vi "Change Count.vi"(0 "connection ID in":refnum<k5>, 2 "Timeout (ms)":i32=40000000, 3 "TxFreqIndex":i32, 4 "TxWaveformStyle":i32, 5 "TxFreqIndex":dbl[](array[numeric])) -> (7 "connection ID out":refnum<k5>)   [LabVIEW 2016]
uses:
  TemperatureMeasure/Thermal_type.vi
panel:
  out "Matched Txfreq":i32[](array[numeric])
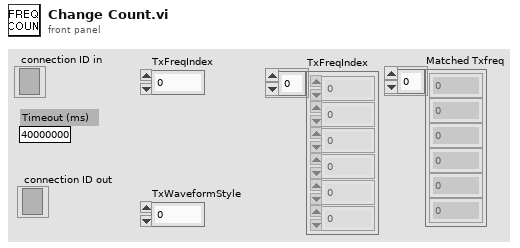
[diagram p1: front panel]
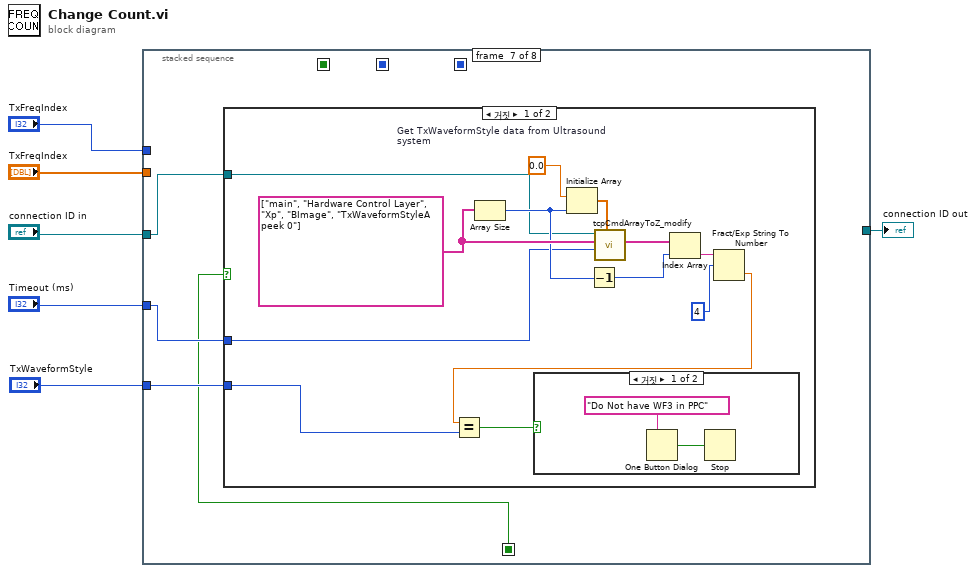
[diagram p0: block diagram]
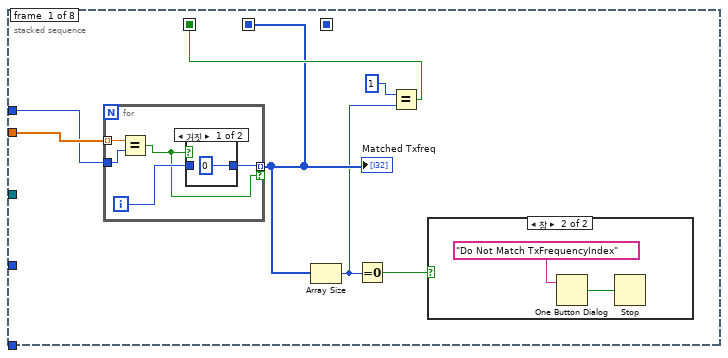
[diagram p2: hidden frame]
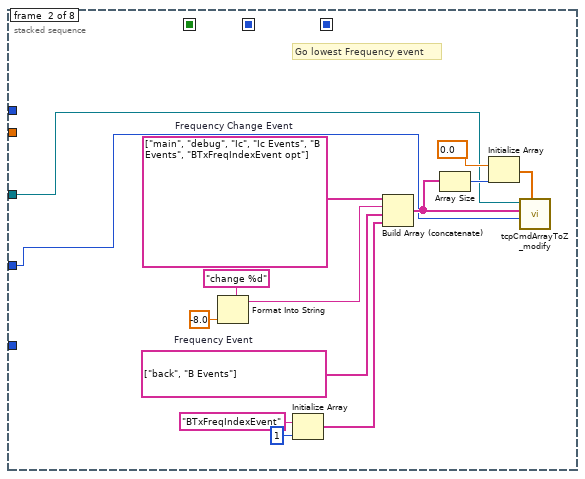
[diagram p5: hidden frame]
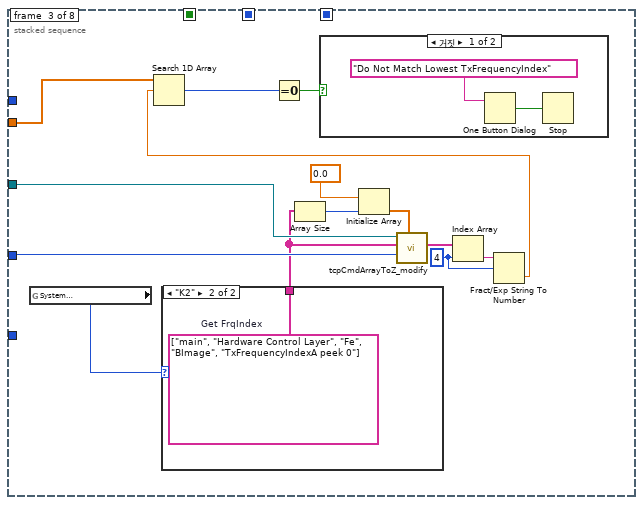
[diagram p6: hidden frame]
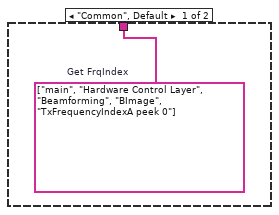
[diagram p7: hidden frame]
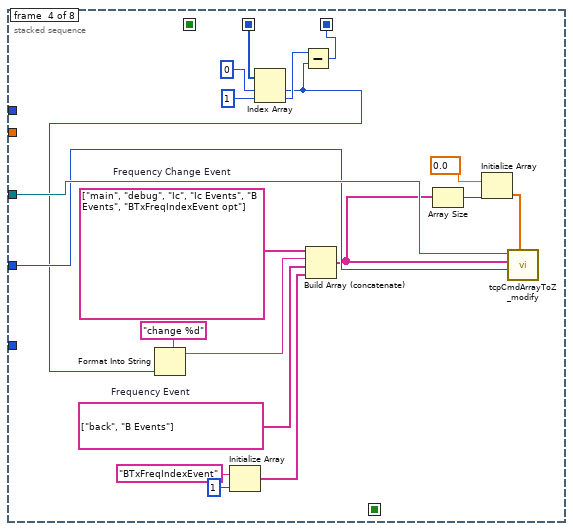
[diagram p9: hidden frame]
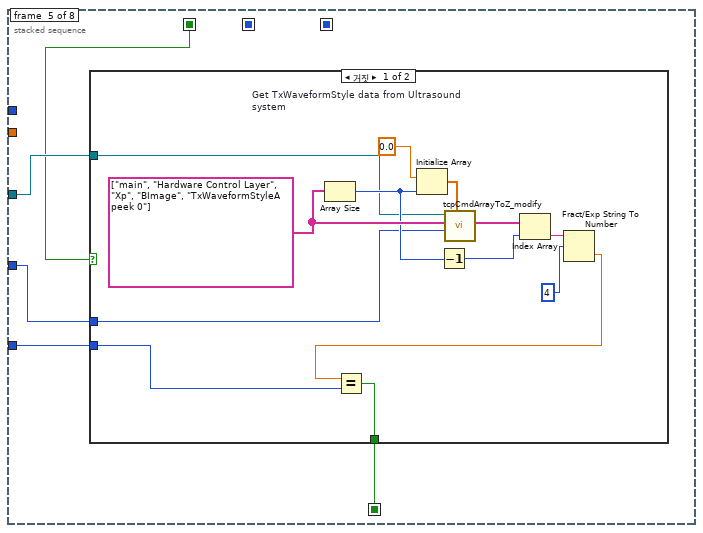
[diagram p10: hidden frame]
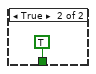
[diagram p11: hidden frame]
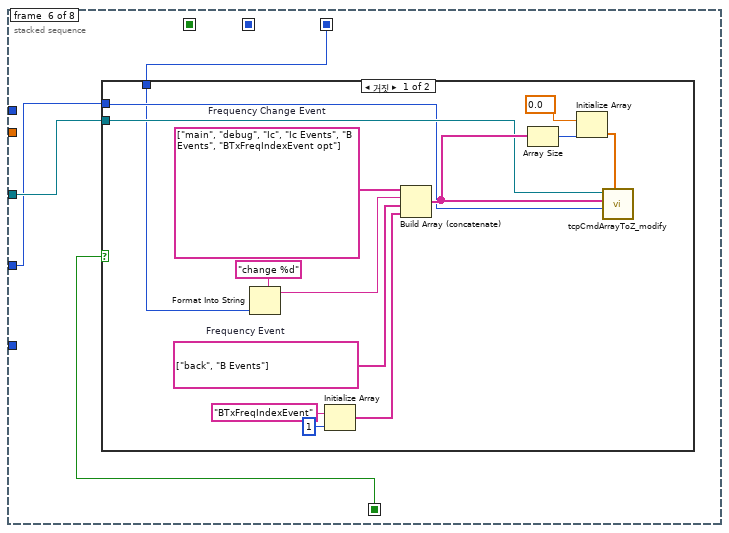
[diagram p12: hidden frame]
diagram:
  n1 = stacked-sequence {
    seq-local: [w10 _ _ _ _ _ _ _] -> [_ _ _ _ w76 _ _ _]
    seq-local: [w8 _ _ _ _ _ _ _] -> [_ _ _ w71 _ _ _ _]
    seq-local: [_ _ _ w56 _ _ _ _] -> [_ _ _ _ _ w94 _ _]
    seq-local: [_ _ _ _ w74 _ _ _] -> [_ _ _ _ _ w93 w112 _]
    tunnel: "TxFreqIndex" -> [w13 _ w42 _ _ _ _ _]
    tunnel: "TxFreqIndex" -> [w12 _ _ _ _ _ _ _]
    tunnel: "Timeout (ms)" -> [_ w24 w43 w72 w77 w95 w113 _]
    tunnel: "connection ID in" -> [_ w25 w44 w73 w78 w96 w111 w130]
    tunnel: [_ _ _ _ _ _ _ w130] -> w2
    tunnel: "TxWaveformStyle" -> [_ _ _ _ w75 _ w114 _]
    frame #0 {
      n2 = for {
        tunnel: w13 -> [w18] mode=indexing
        tunnel: w12 -> [w17]
        tunnel: [w16] -> w8 mode=indexing if=w14
        i -> [w15]
        n3 = Equal?(x=w18, y=w17) -> (x = y?=w14:bool)
        n4 = case shown="거짓" w14 {
          tunnel: [0 w20] -> w16
          tunnel: w15 -> [_ w20]
          frame False {
          }
          frame True {
          }
        }
      }
      "Matched Txfreq" <- w8
      n5 = Array Size(array=w8) -> (size(s)=w7:i32)
      n6 = Equal To 0?(x=w7) -> (x = 0?=w9:bool)
      n7 = Equal?(x=1, y=w7) -> (x = y?=w10:bool)
      n8 = case shown="참" w9 {
        frame False {
        }
        frame True {
          n9 = One Button Dialog(message="Do Not Match TxFrequencyIndex" ("메시지")) -> (true=w21:bool)  [unwired: 1 in]
          n10 = Stop(stop? (T)=w21) -> ()
        }
      }
    }
    frame #1 {
      w27 = string[] ["back", "B Events"]  # Frequency Event
      w31 = string[] ["main", "debug", "Ic", "Ic Events", "B Events", "BTxFreqIndexEvent opt"]  # Frequency Change Event
      # "Go lowest Frequency event"
      n11 = Format Into String(format string="change %d" ("Format String"), -8.0 ("입력 1")) -> (resulting string=w30:string)  [unwired: 2 in, 1 out]
      n12 = Initialize Array("BTxFreqIndexEvent", 1 ("dimension size")) -> (w26:string[])
      n13 = Build Array (concatenate)(w31, w30, w27, w26) -> (w34:string[])
      n14 = Array Size(array=w34) -> (size(s)=w36:i32)
      n15 = Initialize Array(sgl 0.0 ("element"), w36) -> (w33:sgl[])
      n16 = call "tcpCmdArrayToZ_modify.vi"("Delay (sec)"=w33, "Timeout (ms)"=w24, "Command array"=w34, "connection ID in"=w25) -> ()  [unwired: 3 in, 5 out]
    }
    frame #2 {
      w50 = 4 ("index")
      n17 = global read "Thermal_type.vi" "System \nSelection"() -> (w38:enum32{"Common", "Frosk", "Griffin", "K2"})
      n18 = case shown="\"K2\"" w38 {
        tunnel: [w51 w52] -> w37
        frame "Common", Default {
          w51 = string[] ["main", "Hardware Control Layer", "Beamforming", "BImage", "TxFrequencyIndexA peek 0"]  # Get FrqIndex
        }
        frame "K2" {
          w52 = string[] ["main", "Hardware Control Layer", "Fe", "BImage", "TxFrequencyIndexA peek 0"]  # Get FrqIndex
        }
      }
      n19 = Array Size(array=w37) -> (size(s)=w45:i32)
      n20 = Initialize Array(sgl 0.0 ("element"), w45) -> (w47:sgl[])
      n21 = call "tcpCmdArrayToZ_modify.vi"("Delay (sec)"=w47, "Timeout (ms)"=w43, "Command array"=w37, "connection ID in"=w44) -> ("Receive array"=w48:string[])  [unwired: 3 in, 4 out]
      n22 = Index Array(array=w48, index=w50) -> (element=w49:string)
      n23 = Fract/Exp String To Number(string=w49, offset=w50) -> (number=w41:dbl)  [unwired: 2 in, 1 out]
      n24 = Search 1D Array(1D array=w42, element=w41) -> (index of element=w39:i32)  [unwired: 1 in]
      n25 = Equal To 0?(x=w39) -> (x = 0?=w40:bool)
      n26 = case shown="거짓" w40 {
        frame False {
          n27 = One Button Dialog(message="Do Not Match Lowest TxFrequencyIndex" ("메시지")) -> (true=w53:bool)  [unwired: 1 in]
          n28 = Stop(stop? (T)=w53) -> ()
        }
        frame True {
        }
      }
    }
    frame #3 {
      w60 = string[] ["back", "B Events"]  # Frequency Event
      w64 = string[] ["main", "debug", "Ic", "Ic Events", "B Events", "BTxFreqIndexEvent opt"]  # Frequency Change Event
      n29 = Initialize Array("BTxFreqIndexEvent", 1 ("dimension size")) -> (w59:string[])
      n30 = Index Array(array=w71, index #1=0 ("인덱스"), index #2=1 ("인덱스")) -> (element #1=w55:i32, element #2=w57:i32)
      n31 = Format Into String(format string="change %d" ("Format String"), w55) -> (resulting string=w63:string)  [unwired: 2 in, 1 out]
      n32 = Subtract(x=w57, y=w55) -> (x-y=w56:i32)
      n33 = Build Array (concatenate)(w64, w63, w60, w59) -> (w67:string[])
      n34 = Array Size(array=w67) -> (size(s)=w69:i32)
      n35 = Initialize Array(sgl 0.0 ("element"), w69) -> (w66:sgl[])
      n36 = call "tcpCmdArrayToZ_modify.vi"("Delay (sec)"=w66, "Timeout (ms)"=w72, "Command array"=w67, "connection ID in"=w73) -> ()  [unwired: 3 in, 5 out]
    }
    frame #4 {
      n37 = case shown="거짓" w76 {
        tunnel: w78 -> [w83 _]
        tunnel: w77 -> [w82 _]
        tunnel: w75 -> [w81 _]
        tunnel: [w79 TRUE] -> w74
        frame False {
          w91 = string[] ["main", "Hardware Control Layer", "Xp", "BImage", "TxWaveformStyleA peek 0"]  # Get TxWaveformStyle data from Ultrasound system
          n38 = Array Size(array=w91) -> (size(s)=w87:i32)
          n39 = Initialize Array(0.0 ("원소"), w87) -> (w89:dbl[])
          n40 = Decrement(x=w87) -> (x-1=w85:i32)
          n41 = call "tcpCmdArrayToZ_modify.vi"("Delay (sec)"=w89, "Timeout (ms)"=w82, "Command array"=w91, "connection ID in"=w83) -> ("Receive array"=w88:string[])  [unwired: 3 in, 4 out]
          n42 = Index Array(array=w88, index=w85) -> (element=w86:string)
          n43 = Fract/Exp String To Number(string=w86, offset=4 ("오프셋")) -> (number=w80:dbl)  [unwired: 2 in, 1 out]
          n44 = Equal?(x=w80, y=w81) -> (x = y?=w79:bool)
        }
        frame True {
        }
      }
    }
    frame #5 {
      n45 = case shown="거짓" w93 {
        tunnel: w96 -> [w99 _]
        tunnel: w95 -> [w98 _]
        tunnel: w94 -> [w97 _]
        frame False {
          w101 = string[] ["back", "B Events"]  # Frequency Event
          w105 = string[] ["main", "debug", "Ic", "Ic Events", "B Events", "BTxFreqIndexEvent opt"]  # Frequency Change Event
          n46 = Format Into String(format string="change %d" ("Format String"), w97) -> (resulting string=w104:string)  [unwired: 2 in, 1 out]
          n47 = Initialize Array("BTxFreqIndexEvent", 1 ("dimension size")) -> (w100:string[])
          n48 = Build Array (concatenate)(w105, w104, w101, w100) -> (w108:string[])
          n49 = Array Size(array=w108) -> (size(s)=w110:i32)
          n50 = Initialize Array(sgl 0.0 ("element"), w110) -> (w107:sgl[])
          n51 = call "tcpCmdArrayToZ_modify.vi"("Delay (sec)"=w107, "Timeout (ms)"=w98, "Command array"=w108, "connection ID in"=w99) -> ()  [unwired: 3 in, 5 out]
        }
        frame True {
        }
      }
    }
    frame #6 {
      n52 = case shown="거짓" w112 {
        tunnel: w114 -> [w118 _]
        tunnel: w113 -> [w117 _]
        tunnel: w111 -> [w116 _]
        frame False {
          w127 = string[] ["main", "Hardware Control Layer", "Xp", "BImage", "TxWaveformStyleA peek 0"]  # Get TxWaveformStyle data from Ultrasound system
          n53 = Array Size(array=w127) -> (size(s)=w123:i32)
          n54 = Initialize Array(0.0 ("원소"), w123) -> (w125:dbl[])
          n55 = Decrement(x=w123) -> (x-1=w121:i32)
          n56 = call "tcpCmdArrayToZ_modify.vi"("Delay (sec)"=w125, "Timeout (ms)"=w117, "Command array"=w127, "connection ID in"=w116) -> ("Receive array"=w124:string[])  [unwired: 3 in, 4 out]
          n57 = Index Array(array=w124, index=w121) -> (element=w122:string)
          n58 = Fract/Exp String To Number(string=w122, offset=4 ("오프셋")) -> (number=w119:dbl)  [unwired: 2 in, 1 out]
          n59 = Equal?(x=w119, y=w118) -> (x = y?=w115:bool)
          n60 = case shown="거짓" w115 {
            frame False {
              n61 = One Button Dialog(message="Do Not have WF3 in PPC" ("메시지")) -> (true=w128:bool)  [unwired: 1 in]
              n62 = Stop(stop? (T)=w128) -> ()
            }
            frame True {
            }
          }
        }
        frame True {
        }
      }
    }
    frame #7 {
    }
  }
  "connection ID out" <- w2
